vi "Mini projek.vi"() -> ()   [LabVIEW 2016]
uses:
  <vilib>/measure/maspectr.llb/FFT Power Spectrum and PSD for N Chan.vi
  <vilib>/express/express analysis/Spectral/Block/exnSpectralBlock spectral measurements peak poly.vi
  <vilib>/express/express analysis/Spectral/Block/exnSpectralBlock spectral measurements peak DDT.vi
  <vilib>/express/express analysis/Spectral/XNode/ExpressSpectralMeasurementsBlockNode.xnode
  <vilib>/gmath/NI_Gmath.lvlib
  <vilib>/measure/NI_MAPro.lvlib
panel:
  out "Time Domain 2":dynamicdata(graph)
  in  "Stop":bool
  out "Samples Read":i32
  out "Time Domain":waveform(dbl)[](graph)
  out "STFT Spectrogram":dbl[][](graph)
  in  "file path":path
  in  "number of samples/ch (-1: all)":i32=-1
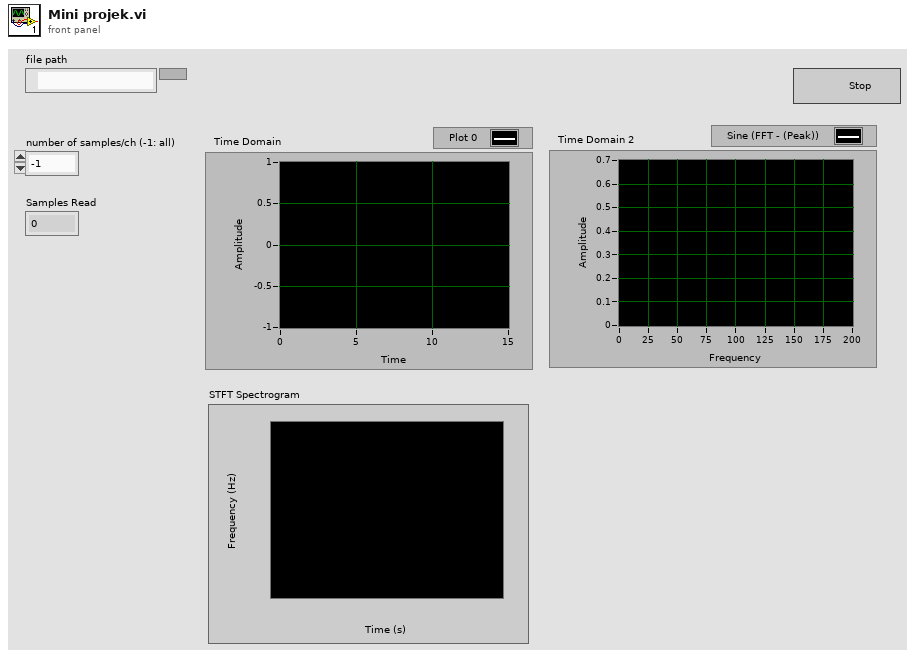
[diagram p1: front panel]
types:
  T1 = cluster{"averaging mode":u16, "weighting mode":u16, "number of averages":u32}
  T2 = cluster{"dB On (F)":bool, "unwrap phase (F)":bool, "convert to degree (F)":bool}
  T3 = cluster{"data[0]":waveform(dbl), "data[1]":waveform(dbl), "data[2]":waveform(dbl), "data[3]":waveform(dbl), "data[4]":waveform(dbl), "data[5]":waveform(dbl), "data[6]":waveform(dbl), "data[7]":waveform(dbl), "data[8]":waveform(dbl)}
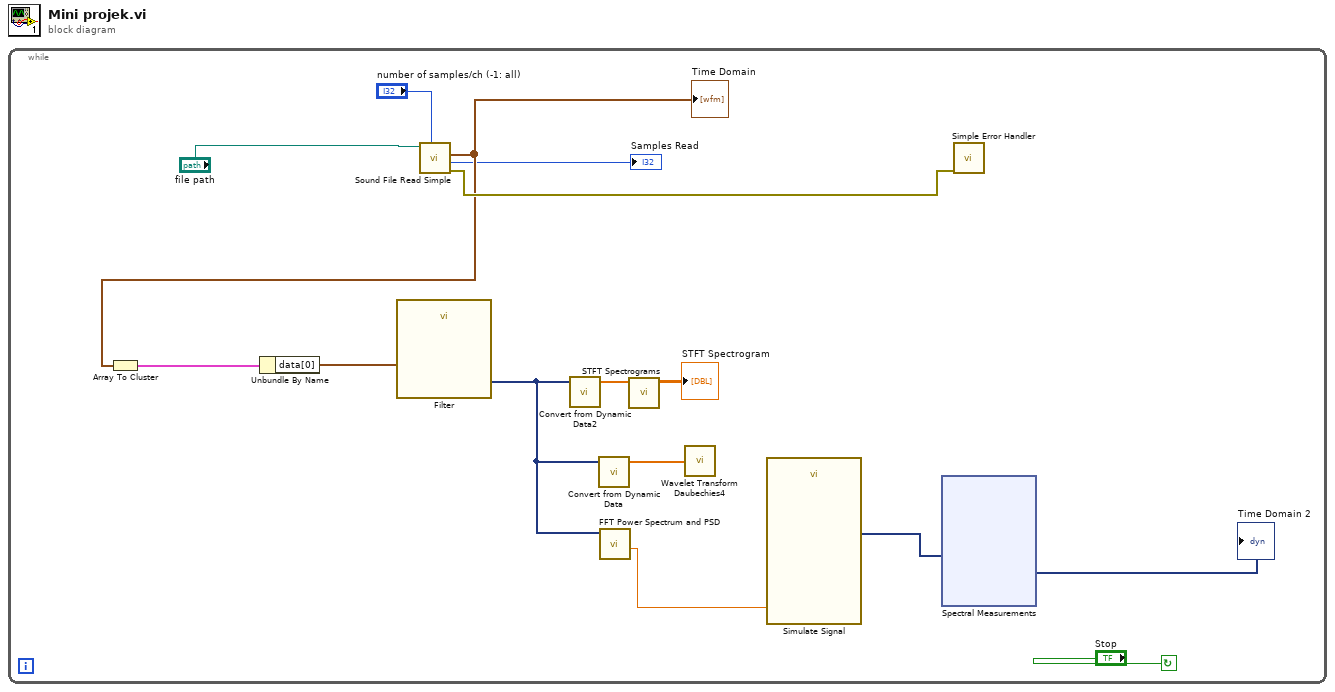
[diagram p0: block diagram]
diagram:
  n1 = while {
    stop <- "Stop" continue-if-true
    n2 = call <vilib>:"Sound File Read Simple.vi"("number of samples/ch (-1: all)"="number of samples/ch (-1: all)", "path"="file path") -> ("error out"=w14:errorcluster, "offset"=→"Samples Read":i32, "data"=w13:waveform(dbl)[])  [unwired: 6 in, 1 out]
    "Time Domain" <- w13
    n3 = Array To Cluster(array=w13) -> (cluster=w9:T3)
    n4 = Unbundle By Name(w9) -> ("data[0]"=w8:waveform(dbl))
    n5 = call "Filter"("Signal"=w8) -> ("Filtered Signal"=w7:dynamicdata)  [unwired: 9 in, 1 out]
    n6 = call "Convert from Dynamic Data2"("Dynamic Data Type"=w7) -> ("Array"=w6:dbl[])  [unwired: 3 in]
    n7 = call "Convert from Dynamic Data"("Dynamic Data Type"=w7) -> ("Array"=w11:dbl[])  [unwired: 3 in]
    n8 = call-poly <vilib>:"FFT Power Spectrum and PSD.vi"("time signals"=w7) -> ("averages completed"=w4:dbl)  [unwired: 7 in, 3 out]
    n9 = call <vilib>:"STFT Spectrograms.vi"("X"=w6) -> ("STFT Spectrogram {X}"=→"STFT Spectrogram":dbl[][])  [unwired: 9 in, 1 out]
    n10 = call <vilib>:"Wavelet Transform Daubechies4.vi"("X"=w11) -> ()  [unwired: 2 out]
    n11 = call "Simulate Signal"("Frequency"=w4) -> ("Sine"=w2:dynamicdata)  [unwired: 13 in, 1 out]
    n12 = xnode "Spectral Measurements"("Signals"=w2) -> ("FFT - (Peak)"=→"Time Domain 2":dynamicdata)  [unwired: 1 in, 2 out]
    n13 = call <vilib>:"Simple Error Handler.vi"("error in (no error)"=w14) -> ()  [unwired: 4 in, 5 out]
  }
